vi "Notify.vi"(8 "Error In":errorcluster, 11 "reference in":refnum<class "CommunicationModule.lvclass">) -> (0 "Error Out":errorcluster, 3 "reference out":refnum<class "CommunicationModule.lvclass">)   [LabVIEW 2024, in "CommunicationModule.lvclass"]
uses:
  CommunicationModule.lvclass
  CommunicationModule.lvclass/CommunicationModule.ctl
  C:/Users/burakkorkmaz/Desktop/Leveling/labview-design-patterns/Observer Pattern/CommunicationModule/CommunicationModule.lvclass
  C:/Users/burakkorkmaz/Desktop/Leveling/labview-design-patterns/Observer Pattern/IObservable/IObservable.lvclass
  IObserver/IObserver.lvclass
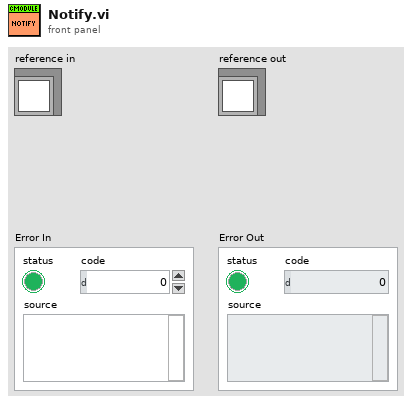
[diagram p1: front panel]
types:
  T1 = typedef "CommunicationModule.lvclass/ObjectAttributes.ctl" = cluster{"ObserverList":refnum<class "IObserver.lvclass">[]}
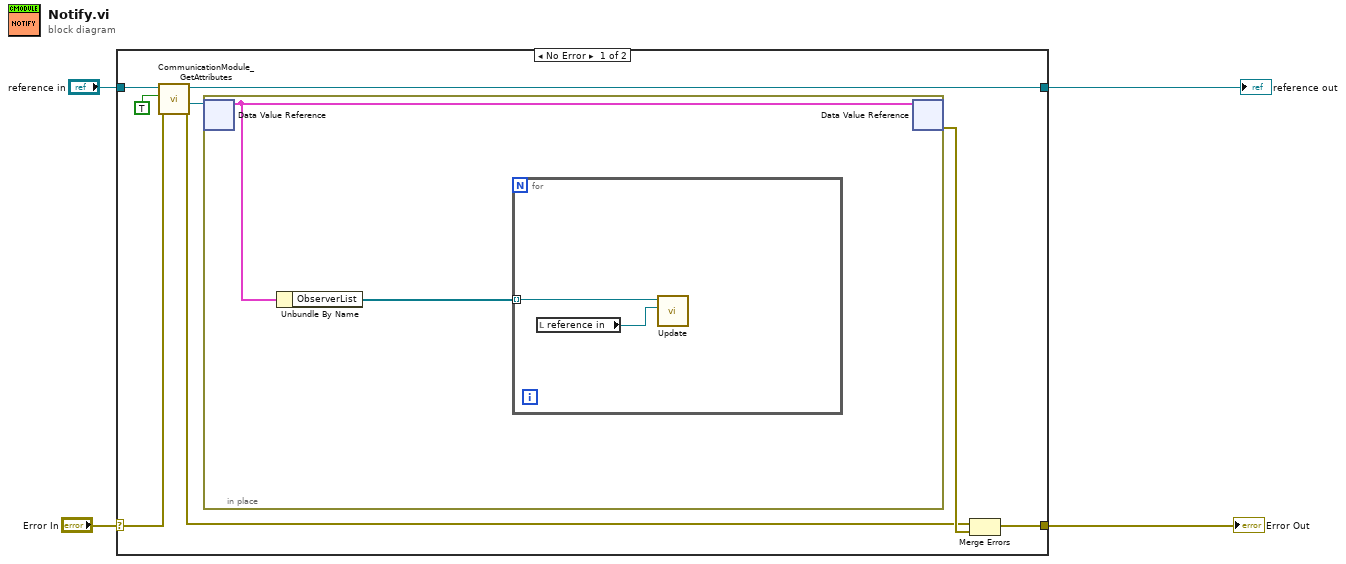
[diagram p0: block diagram]
diagram:
  n1 = case shown="No Error" "Error In" {
    selector: "Error In" -> [w11 w18]
    tunnel: [w8 w18] -> w3
    tunnel: [w9 w17] -> w1
    tunnel: "reference in" -> [w12 w17]
    frame No Error {
      n2 = call "CommunicationModule_GetAttributes.vi"("Error In"=w11, "OnlyGetDvrReference(False)"=TRUE, "reference in"=w12) -> ("Error Out"=w6:errorcluster, "DataRef"=w7:refnum<data-value>, "reference out"=w9:refnum<class "CommunicationModule.lvclass">)  [unwired: 5 in, 1 out]
      n3 = in-place {
        n4 = in-place-dvr #1(w7) -> (w14:T1)  [unwired: 1 out]
        n5 = Unbundle By Name(w14) -> ("ObserverList"=w13:refnum<class "IObserver.lvclass">[])
        n6 = for {
          tunnel: w13 -> [w16] mode=indexing
          n7 = local read "reference in"() -> (w15:refnum<class "CommunicationModule.lvclass">)
          n8 = call-dynamic "Update.vi"("IObservable"=w15, "object in"=w16) -> ()  [unwired: 8 in, 2 out]
        }
        n9 = in-place-dvr #1(w14) -> (w10:errorcluster)  [unwired: 1 out]
      }
      n10 = Merge Errors(w6, w10) -> (w8:errorcluster)
    }
    frame Error {
    }
  }
  "Error Out" <- w3
  "reference out" <- w1
